vi "Obtain Request Events.vi"(8 "error in":errorcluster, 10 "Create New? (F)":bool) -> (0 "error out":errorcluster, 2 "DeviceManager Request Events":T1)   [LabVIEW 2023, in "horiba.lvlib" / "DeviceManager.lvlib"]
doc: "This VI Obtains/Creates the Requests events that will be used for other modules to communicate with the module that owns this VI. These Requests events will be accessed only via Public API methods for this module.\n\n<b>NOTE</b>: The contents of this VI are automatically generated and modified by the <b>Tools > DQMH Consortium > DQMH</b> utilities. Consider using those utilities instead of making your own modifications to this VI.\n_____\nBased on DQMH Project Template 7.0.0.1280."
uses:
  DeviceManager.lvlib
  Request Events--cluster.ctl
  Stop Argument--cluster.ctl
  Show Panel Argument--cluster.ctl
  Hide Panel Argument--cluster.ctl
  Get Module Execution Status Argument--cluster.ctl
  Show Diagram Argument--cluster.ctl
  StartICL Argument--cluster.ctl
  OpenWebSocketCommunication Argument--cluster.ctl
  OpenWebSocketCommunication (Reply Payload)--cluster.ctl
  ICLstartNotification Argument--cluster.ctl
  ICLshutdown Argument--cluster.ctl
  SendJSONandAskForReply Argument--cluster.ctl
  SendJSONandAskForReply (Reply Payload)--cluster.ctl
  DiscoverDevices Argument--cluster.ctl
  DiscoverDevices (Reply Payload)--cluster.ctl
  Mono/Monochromator.lvclass
  CCD/CCD.lvclass
  SCD/SCD.lvclass
  DevicesList Argument--cluster.ctl
  DevicesList (Reply Payload)--cluster.ctl
panel:
  # "NOTE: The contents of this VI are automatically generated and modified by the Tools > DQMH Consortium > DQMH utilities. Consider using those utilities instead of making your own modifications to this VI."
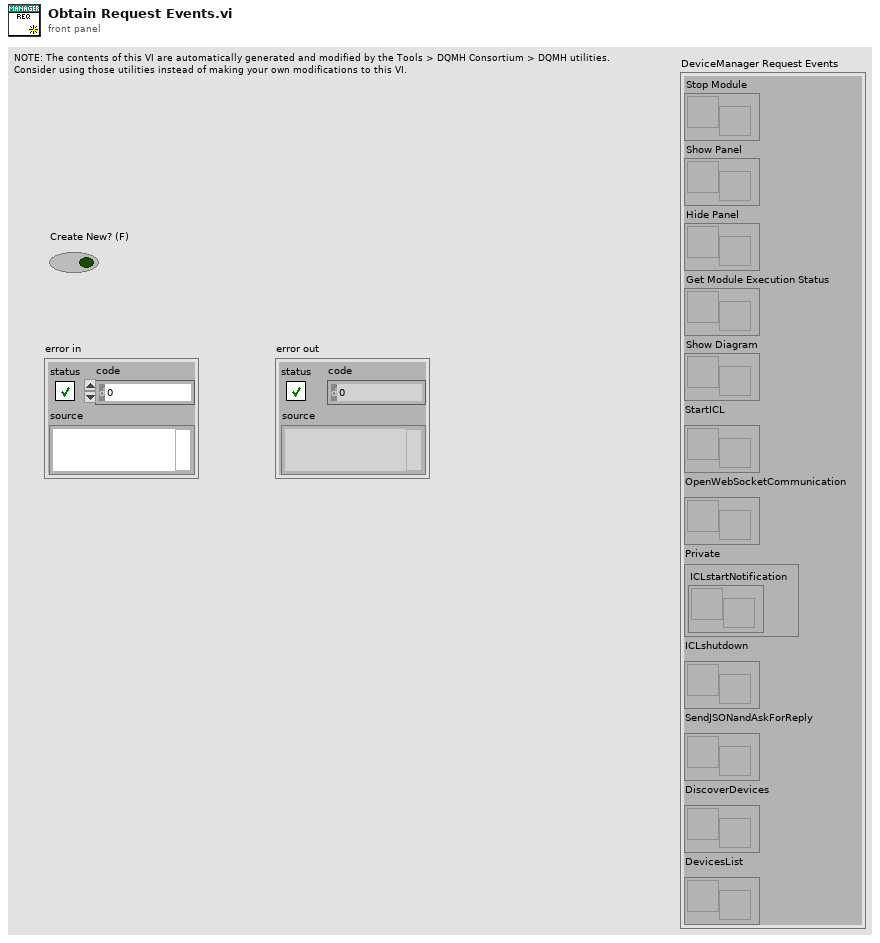
[diagram p1: front panel]
types:
  T1 = typedef "horiba.lvlib/DeviceManager.lvlib/Request Events--cluster.ctl" = cluster{"Stop Module":refnum<user-event>, "Show Panel":refnum<user-event>, "Hide Panel":refnum<user-event>, "Get Module Execution Status":refnum<user-event>, "Show Diagram":refnum<user-event>, "StartICL":refnum<user-event>, "OpenWebSocketCommunication":refnum<user-event>, "Private":cluster{"ICLstartNotification":refnum<user-event>}, "ICLshutdown":refnum<user-event>, "SendJSONandAskForReply":refnum<user-event>, "DiscoverDevices":refnum<user-event>, "DevicesList":refnum<user-event>}
  T2 = typedef "horiba.lvlib/DeviceManager.lvlib/DevicesList Argument--cluster.ctl" = cluster{"Time out [ms]":i32, "Wait Notifier":refnum<notifier>, "wait for reply":bool}
  T3 = typedef "horiba.lvlib/DeviceManager.lvlib/DiscoverDevices Argument--cluster.ctl" = cluster{"Wait Notifier":refnum<notifier>, "wait for reply":bool, "timeout for discovering devices [ms]":i32}
  T4 = typedef "horiba.lvlib/DeviceManager.lvlib/SendJSONandAskForReply Argument--cluster.ctl" = cluster{"JSON to be sent":string, "Delay between send and receive [ms]":i32, "Wait Notifier":refnum<notifier>, "wait for reply":bool}
  T5 = typedef "horiba.lvlib/DeviceManager.lvlib/ICLshutdown Argument--cluster.ctl" = cluster{"Boolean":bool}
  T6 = typedef "horiba.lvlib/DeviceManager.lvlib/ICLstartNotification Argument--cluster.ctl" = cluster{"Boolean":bool}
  T7 = typedef "horiba.lvlib/DeviceManager.lvlib/OpenWebSocketCommunication Argument--cluster.ctl" = cluster{"WS Server IP":string, "WS Server Port":string, "timeout opening [ms]":i32, "timeout hand shake [ms]":i32, "Wait Notifier":refnum<notifier>, "wait for reply":bool}
  T8 = typedef "horiba.lvlib/DeviceManager.lvlib/StartICL Argument--cluster.ctl" = cluster{"show ICL for debugging":bool}
  T9 = typedef "horiba.lvlib/DeviceManager.lvlib/Hide Panel Argument--cluster.ctl" = cluster{"Hide Panel?":bool}
  T10 = typedef "horiba.lvlib/DeviceManager.lvlib/Show Panel Argument--cluster.ctl" = cluster{"Show Panel?":bool}
  T11 = typedef "horiba.lvlib/DeviceManager.lvlib/Show Diagram Argument--cluster.ctl" = cluster{"Debug?":bool}
  T12 = typedef "horiba.lvlib/DeviceManager.lvlib/Get Module Execution Status Argument--cluster.ctl" = cluster{"Running?":bool}
  T13 = typedef "horiba.lvlib/DeviceManager.lvlib/Stop Argument--cluster.ctl" = cluster{"Origin":string, "Exit via Stop Module Req?":bool, "Wait for Module to stop?":bool}
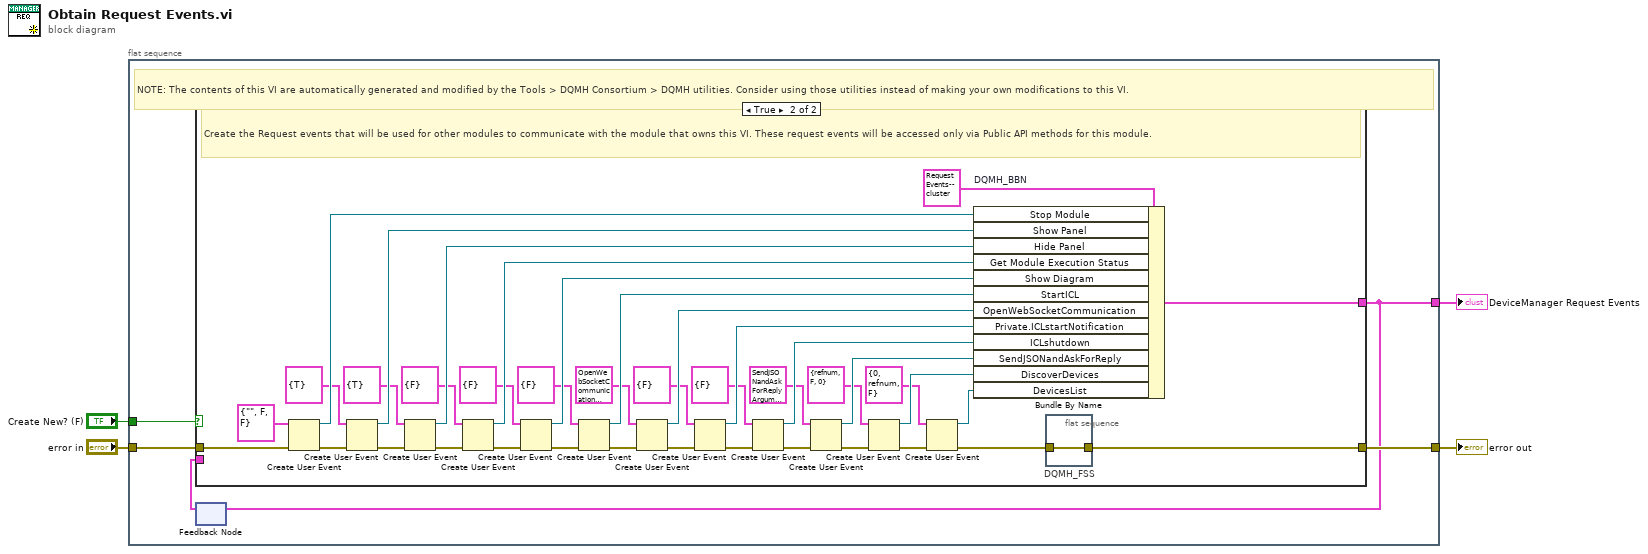
[diagram p0: block diagram]
diagram:
  n1 = flat-sequence {
    tunnel: [w9] -> w4
    tunnel: "error in" -> [w8]
    tunnel: [w6] -> w2
    tunnel: "Create New? (F)" -> [w5]
    frame #0 {
      # "NOTE: The contents of this VI are automatically generated and modified by the Tools > DQMH Consortium > DQMH utilities. Consider using those utilities instead of making your own modifications to this VI."
      n2 = feedback #1() -> (w7:T1)  [unwired: 1 in]
      n3 = case shown="True" w5 {
        tunnel: [w10 w41] -> w9
        tunnel: w8 -> [w10 w51]
        tunnel: [w11 w48] -> w6
        tunnel: w7 -> [w11 _]
        frame False {
          # "Obtain the Request events that were created in a previous call to this VI."
        }
        frame True {
          # "Create the Request events that will be used for other modules to communicate with the module that owns this VI. These request events will be accessed only via Public API methods for this module."
          n4 = Create User Event(user event datatype=T13 {"Origin"="", "Exit via Stop Module Req?"=FALSE, "Wait for Module to stop?"=FALSE} ("Stop Argument"), error in=w51) -> (user event=w49:refnum<user-event>, error out=w46:errorcluster)
          n5 = Create User Event(user event datatype=T10 {"Show Panel?"=TRUE} ("Show Panel Argument"), error in=w46) -> (user event=w45:refnum<user-event>, error out=w44:errorcluster)
          n6 = Create User Event(user event datatype=T9 {"Hide Panel?"=TRUE} ("Hide Panel Argument"), error in=w44) -> (user event=w43:refnum<user-event>, error out=w42:errorcluster)
          n7 = Create User Event(user event datatype=T12 {"Running?"=FALSE} ("Get Module Execution Status Argument"), error in=w42) -> (user event=w39:refnum<user-event>, error out=w40:errorcluster)
          n8 = Create User Event(user event datatype=T11 {"Debug?"=FALSE} ("Show Diagram Argument"), error in=w40) -> (user event=w36:refnum<user-event>, error out=w37:errorcluster)
          n9 = Create User Event(user event datatype=T8 {"show ICL for debugging"=FALSE} ("StartICL Argument"), error in=w37) -> (user event=w31:refnum<user-event>, error out=w32:errorcluster)
          n10 = Create User Event(user event datatype=T7 {"WS Server IP"="ws://127.0.0.1", "WS Server Port"="25010", "timeout opening [ms]"=5000, "timeout hand shake [ms]"=5000, "Wait Notifier"=refnum, "wait for reply"=FALSE} ("OpenWebSocketCommunication Argument"), error in=w32) -> (user event=w28:refnum<user-event>, error out=w29:errorcluster)
          n11 = Create User Event(user event datatype=T6 {"Boolean"=FALSE} ("ICLstartNotification Argument"), error in=w29) -> (user event=w25:refnum<user-event>, error out=w26:errorcluster)
          n12 = Create User Event(user event datatype=T5 {"Boolean"=FALSE} ("ICLshutdown Argument"), error in=w26) -> (user event=w22:refnum<user-event>, error out=w23:errorcluster)
          n13 = Create User Event(user event datatype=T4 {"JSON to be sent"="{\"id\":1234, \"command\":\"icl_info\"}", "Delay between send and receive [ms]"=0, "Wait Notifier"=refnum, "wait for reply"=FALSE} ("SendJSONandAskForReply Argument"), error in=w23) -> (user event=w19:refnum<user-event>, error out=w20:errorcluster)
          n14 = Create User Event(user event datatype=T3 {"Wait Notifier"=refnum, "wait for reply"=FALSE, "timeout for discovering devices [ms]"=0} ("DiscoverDevices Argument"), error in=w20) -> (user event=w16:refnum<user-event>, error out=w17:errorcluster)
          n15 = Create User Event(user event datatype=T2 {"Time out [ms]"=0, "Wait Notifier"=refnum, "wait for reply"=FALSE} ("DevicesList Argument"), error in=w17) -> (user event=w13:refnum<user-event>, error out=w14:errorcluster)
          n16 = Bundle By Name "DQMH_BBN"(cluster=T1 {"Stop Module"=refnum, "Show Panel"=refnum, "Hide Panel"=refnum, "Get Module Execution Status"=refnum, "Show Diagram"=refnum, "StartICL"=refnum, "OpenWebSocketCommunication"=refnum, "Private"={"ICLstartNotification"=refnum}, "ICLshutdown"=refnum, "SendJSONandAskForReply"=refnum, "DiscoverDevices"=refnum, "DevicesList"=refnum} ("output cluster"), "Stop Module"=w49, "Show Panel"=w45, "Hide Panel"=w43, "Get Module Execution Status"=w39, "Show Diagram"=w36, "StartICL"=w31, "OpenWebSocketCommunication"=w28, "Private.ICLstartNotification"=w25, "ICLshutdown"=w22, "SendJSONandAskForReply"=w19, "DiscoverDevices"=w16, "DevicesList"=w13) -> (w48:T1)
          n17 = flat-sequence "DQMH_FSS" {
            tunnel: w14 -> [w52]
            tunnel: [w52] -> w41
            frame #0 {
            }
          }
        }
      }
      n18 = feedback-in #1(w6) -> ()
    }
  }
  "DeviceManager Request Events" <- w2
  "error out" <- w4
